vi "AB_Engine_DLL_CopyHeaderFiles.vi"(8 "error in (no error)":errorcluster, 10 "Preview?":bool, 11 "Path":path) -> (0 "error out":errorcluster, 3 "GeneratedFiles":path[](array[path]))   [LabVIEW 2020]
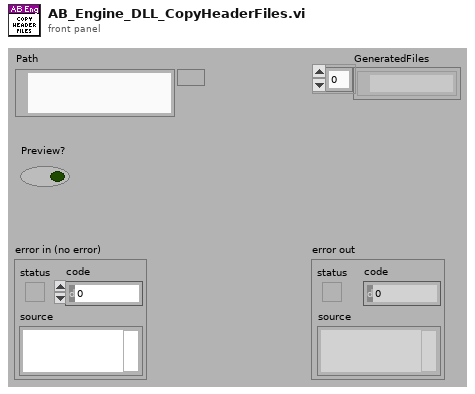
[diagram p1: front panel]
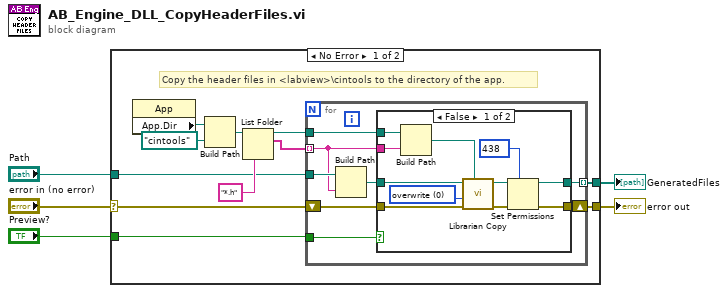
[diagram p0: block diagram]
diagram:
  n1 = case shown="No Error" "error in (no error)" {
    selector: "error in (no error)" -> [w11 w38]
    tunnel: [w10 w38] -> w4
    tunnel: [w9 _] -> w3
    tunnel: "Preview?" -> [w7 _]
    tunnel: "Path" -> [w6 _]
    frame No Error {
      # "Copy the header files in <labview>\\cintools to the directory of the app."
      n2 = property class="App"() -> ("App.Dir"=w15:path)  [unwired: 2 in, 2 out]
      n3 = Build Path(base path=w15, name or relative path=path "cintools") -> (appended path=w14:path)
      n4 = List Folder(path=w14, pattern="*.h") -> (path out=w12:path, filenames=w8:string[])  [unwired: 2 in, 2 out]
      n5 = for {
        tunnel: w12 -> [w18]
        tunnel: w8 -> [w17] mode=indexing
        tunnel: w6 -> [w24]
        shift-right: [w21] -> w10
        shift-left: w11 -> [w22]
        tunnel: [w20] -> w9 mode=indexing
        tunnel: w7 -> [w19]
        n6 = Build Path(base path=w24, name or relative path=w17) -> (appended path=w23:path)
        n7 = case shown="False" w19 {
          tunnel: w23 -> [w35 w37]
          tunnel: w22 -> [w30 w36]
          tunnel: [w29 w36] -> w21
          tunnel: [w28 w37] -> w20
          tunnel: w18 -> [w27 _]
          tunnel: w17 -> [w26 _]
          frame False {
            w34 = u16 0 items=["overwrite", "ask first", "don't overwrite"] ("overwrite")
            n8 = Build Path(base path=w27, name or relative path=w26) -> (appended path=w25:path)
            n9 = call <vilib>:"Librarian Copy.vi"("source"=w25, "error in (no error)"=w30, "overwrite"=w34, "destination"=w35) -> ("error out"=w33:errorcluster, "dup destination"=w32:path)  [unwired: 6 in]
            n10 = Set Permissions(7:i16 438 ("permissions"), 8:w33, 11:w32) -> (0:w29:errorcluster, 3:w28:path)  [unwired: 2 in]
          }
          frame True {
            # "Only build list of files if preview."
          }
        }
      }
    }
    frame Error {
    }
  }
  "error out" <- w4
  "GeneratedFiles" <- w3
